vi "cruce por cero adders.vi"(9 "Vin Asic Real":dbl[](array[numeric])=[0.051, 0.101, 0.201], 10 "Volt LLTH":dbl[][][](array[numeric]), 11 "Volt HLTH":dbl[][][](array[numeric])) -> (0 "Volt LLTH Corregido":dbl[][][](array[numeric]), 1 "Cruce por 0 Salida b LLTH":dbl[][](array[numeric]), 2 "Cruce por 0 Salida a HLTH":dbl[][](array[numeric]), 3 "Volt HLTH Corregido":dbl[][][](array[numeric]))   [LabVIEW 2019]
uses:
  <vilib>/Analysis/6fits.llb/Curve Fitting Criteria.ctl
  <vilib>/Analysis/NI_AALPro.lvlib
panel:
  # "MODE"
  # "channel"
  # "VIN\nMODE\nCHANNEL"
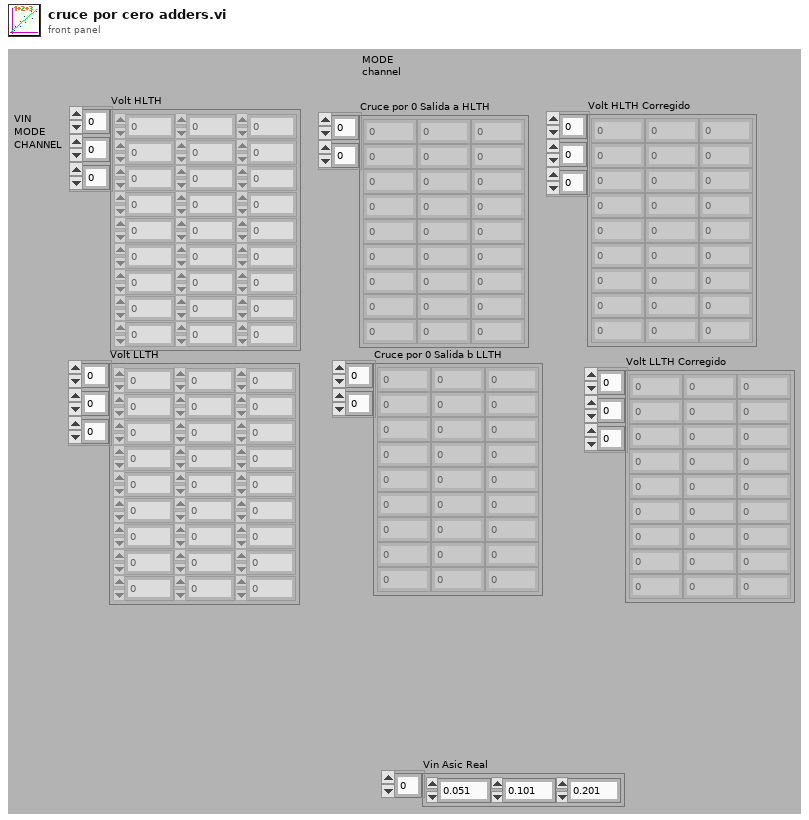
[diagram p1: front panel]
types:
  T1 = typedef "NI_AALPro.lvlib/Curve Fitting Criteria.ctl" = u16
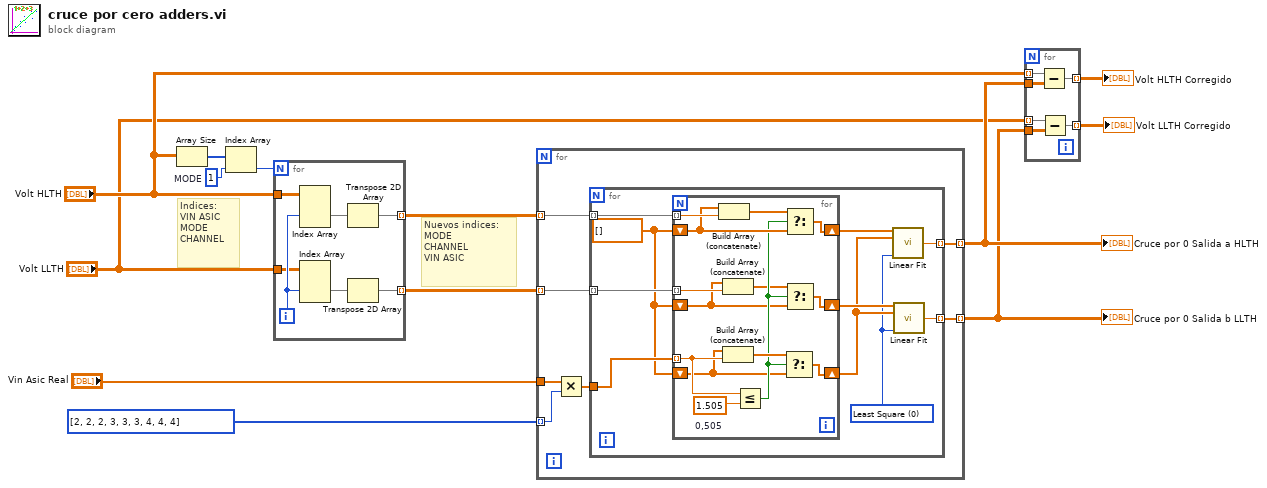
[diagram p0: block diagram]
diagram:
  w12 = 1  # MODE
  # "Indices:\nVIN ASIC\nMODE\nCHANNEL"
  # "Nuevos indices:\nMODE\nCHANNEL\nVIN ASIC"
  n1 = Array Size(array="Volt HLTH") -> (size(s)=w13:i32[])
  n2 = Index Array(array=w13, index=w12) -> (element=w11:i32)
  n3 = for {
    N: w11 -> [_]
    tunnel: "Volt HLTH" -> [w20]
    tunnel: [w18] -> w8 mode=indexing
    tunnel: "Volt LLTH" -> [w15]
    tunnel: [w14] -> w4 mode=indexing
    i -> [w16]
    n4 = Index Array(array=w20, index (dim 1)=w16) -> (element=w19:dbl[][])  [unwired: 2 in]
    n5 = Index Array(array=w15, index (dim 1)=w16) -> (element=w17:dbl[][])  [unwired: 2 in]
    n6 = Transpose 2D Array(2D array=w19) -> (transposed array=w18:dbl[][])
    n7 = Transpose 2D Array(2D array=w17) -> (transposed array=w14:dbl[][])
  }
  n8 = for {
    tunnel: w8 -> [w27] mode=indexing
    tunnel: i32[] [2, 2, 2, 3, 3, 3, 4, 4, 4] -> [w25] mode=indexing
    tunnel: "Vin Asic Real" -> [w26]
    tunnel: [w23] -> w7 mode=indexing
    tunnel: w4 -> [w22] mode=indexing
    tunnel: [w21] -> w3 mode=indexing
    n9 = Multiply(x=w26, y=w25) -> (x*y=w24:dbl[])
    n10 = for {
      tunnel: w27 -> [w36] mode=indexing
      tunnel: w24 -> [w35]
      tunnel: [w37] -> w23 mode=indexing
      tunnel: w22 -> [w33] mode=indexing
      tunnel: [w29] -> w21 mode=indexing
      w32 = dbl[] []
      w28 = T1 0 items=["Least Square", "Least Absolute Residual", "Bisquare"] ("method")
      n11 = for {
        tunnel: w36 -> [w45] mode=indexing
        tunnel: w35 -> [w46] mode=indexing
        shift-right: [w50] -> w34
        shift-left: w32 -> [w44]
        shift-right: [w47] -> w30
        shift-left: w32 -> [w42]
        tunnel: w33 -> [w41] mode=indexing
        shift-right: [w39] -> w31
        shift-left: w32 -> [w38]
        w51 = 1.505  # 0,505
        n12 = Build Array (concatenate)(w44, w45) -> (w49:dbl[])
        n13 = Build Array (concatenate)(w38, w41) -> (w40:dbl[])
        n14 = Build Array (concatenate)(w42, w46) -> (w48:dbl[])
        n15 = Less Or Equal?(x=w46, y=w51) -> (x <= y?=w43:bool)
        n16 = Select(t=w48, s=w43, f=w42) -> (s? t:f=w47:dbl[])
        n17 = Select(t=w49, s=w43, f=w44) -> (s? t:f=w50:dbl[])
        n18 = Select(t=w40, s=w43, f=w38) -> (s? t:f=w39:dbl[])
      }
      n19 = call <vilib>:"Linear Fit.vi"("Y"=w34, "X"=w30, "method"=w28) -> ("intercept"=w37:dbl)  [unwired: 8 in, 4 out]
      n20 = call <vilib>:"Linear Fit.vi"("Y"=w31, "X"=w30, "method"=w28) -> ("intercept"=w29:dbl)  [unwired: 8 in, 4 out]
    }
  }
  "Cruce por 0 Salida a HLTH" <- w7
  "Cruce por 0 Salida b LLTH" <- w3
  n21 = for {
    tunnel: "Volt HLTH" -> [w57] mode=indexing
    tunnel: w7 -> [w56]
    tunnel: [w55] -> w6 mode=indexing
    tunnel: w3 -> [w54]
    tunnel: "Volt LLTH" -> [w53] mode=indexing
    tunnel: [w52] -> w1 mode=indexing
    n22 = Subtract(x=w57, y=w56) -> (x-y=w55:dbl[][])
    n23 = Subtract(x=w53, y=w54) -> (x-y=w52:dbl[][])
  }
  "Volt HLTH Corregido" <- w6
  "Volt LLTH Corregido" <- w1
